vi "Add Children to End.vi"(8 "error in (no error)":errorcluster, 10 "Children":refnum<data-value>[](array[refnum]), 11 "NodeRef In":refnum<data-value>) -> (0 "error out":errorcluster, 3 "NodeRef":refnum<data-value>)   [LabVIEW 2020, in "PicoG-ParserLexer.lvlib" / "Node.lvclass"]
uses:
  Node.lvclass
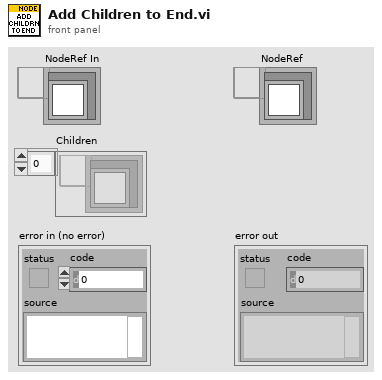
[diagram p1: front panel]
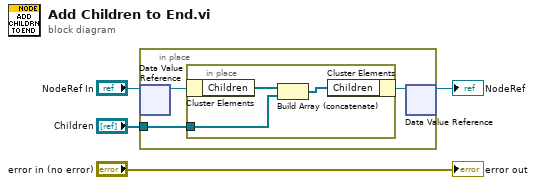
[diagram p0: block diagram]
diagram:
  n1 = in-place {
    in-place-border: "Children" -> [w6]
    n2 = in-place-dvr #1("NodeRef In") -> (w7:refnum<class "Node.lvclass">)  [unwired: 1 out]
    n3 = in-place {
      in-place-border: w6 -> [w10]
      n4 = in-place-cluster #2(w7) -> ("Children"=w9:refnum<data-value>[])
      n5 = Build Array (concatenate)(w9, w10) -> (w8:refnum<data-value>[])
      n6 = in-place-cluster #2("Children"=w8) -> (w5:refnum<class "Node.lvclass">)
    }
    n7 = in-place-dvr #1(w5) -> (→"NodeRef":refnum<data-value>)  [unwired: 1 out]
  }
  "error out" <- "error in (no error)"
